vi "Write.vi"(8 "error in":errorcluster, 9 "Producer Ch":T2, 10 "Producer Control":T1, 11 "Cycler Cluster.lvclass":refnum<class "Power Supply Cluster.lvclass">) -> (0 "error out":errorcluster, 3 "output cluster":refnum<class "Power Supply Cluster.lvclass">)   [LabVIEW 2023, in "Power Supply Cluster.lvclass"]
uses:
  Power Supply Cluster.lvclass
  6bfc6677-cd67-4f2d-afef-839dec9218ce.vi
  74f11eb1-9425-41af-a169-6608e4aa6674.vi
  Producer Ch Array.ctl
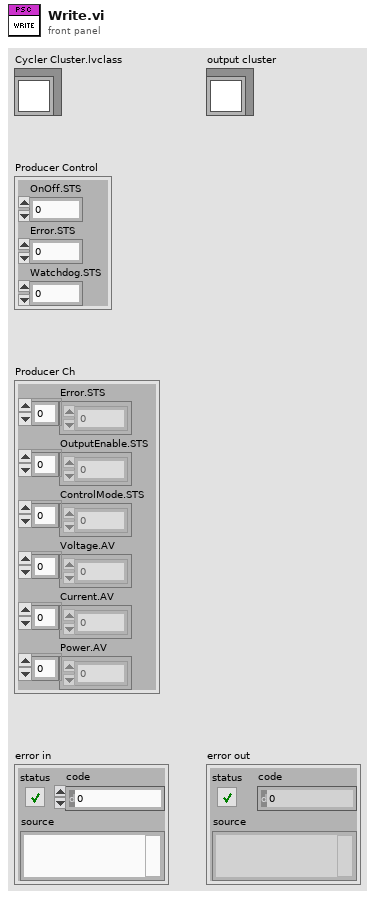
[diagram p1: front panel]
types:
  T1 = cluster{"OnOff.STS":i32, "Error.STS":i32, "Watchdog.STS":i32}
  T2 = typedef "Power Supply Cluster.lvclass/Producer Ch Array.ctl" = cluster{"Error.STS":i32[], "OutputEnable.STS":i32[], "ControlMode.STS":u16[], "Voltage.AV":dbl[], "Current.AV":dbl[], "Power.AV":dbl[]}
  T3 = cluster{"Error.STS":i32, "OutputEnable.STS":i32, "ControlMode.STS":u16, "Voltage.AV":dbl, "Current.AV":dbl, "Power.AV":dbl}
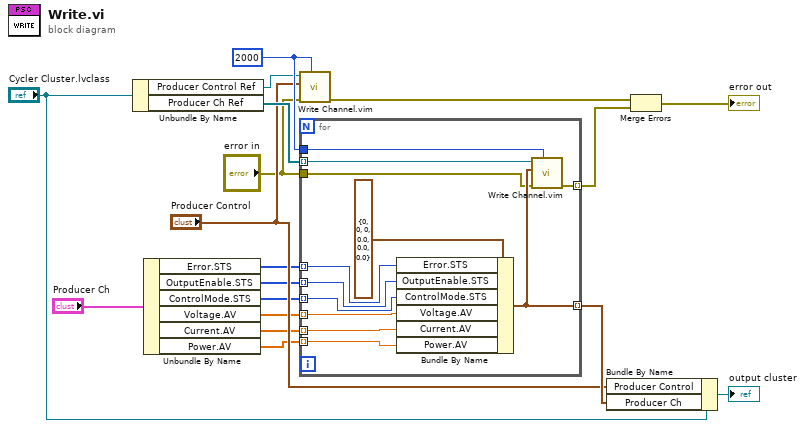
[diagram p0: block diagram]
diagram:
  w14 = 2000 ("Timeout (ms)")
  n1 = Unbundle By Name("Cycler Cluster.lvclass") -> ("Producer Control Ref"=w13:refnum<k21>, "Producer Ch Ref"=w15:refnum<k21>[])
  n2 = Unbundle By Name("Producer Ch") -> ("Error.STS"=w6:i32[], "OutputEnable.STS"=w5:i32[], "ControlMode.STS"=w4:u16[], "Voltage.AV"=w3:dbl[], "Current.AV"=w2:dbl[], "Power.AV"=w1:dbl[])
  n3 = call "Write Channel.vim"("Timeout (ms)"=w14, "error in"="error in", "Data in"="Producer Control", "ADAS HIL Channel in"=w13) -> ("error out"=w9:errorcluster)  [unwired: 5 in, 2 out]
  n4 = for {
    tunnel: [w29] -> w12 mode=indexing
    tunnel: "error in" -> [w28]
    tunnel: [w27] -> w8 mode=indexing
    tunnel: w15 -> [w26] mode=indexing
    tunnel: w14 -> [w25]
    tunnel: w6 -> [w24] mode=indexing
    tunnel: w5 -> [w23] mode=indexing
    tunnel: w4 -> [w22] mode=indexing
    tunnel: w3 -> [w21] mode=indexing
    tunnel: w2 -> [w20] mode=indexing
    tunnel: w1 -> [w19] mode=indexing
    n5 = Bundle By Name(cluster=T3 {"Error.STS"=0, "OutputEnable.STS"=0, "ControlMode.STS"=0, "Voltage.AV"=0.0, "Current.AV"=0.0, "Power.AV"=0.0} ("Producer Ch"), "Error.STS"=w24, "OutputEnable.STS"=w23, "ControlMode.STS"=w22, "Voltage.AV"=w21, "Current.AV"=w20, "Power.AV"=w19) -> (w29:T3)
    n6 = call "Write Channel.vim"("Timeout (ms)"=w25, "error in"=w28, "Data in"=w29, "ADAS HIL Channel in"=w26) -> ("error out"=w27:errorcluster)  [unwired: 5 in, 2 out]
  }
  n7 = Bundle By Name(cluster="Cycler Cluster.lvclass", "Producer Control"="Producer Control", "Producer Ch"=w12) -> (→"output cluster":refnum<class "Power Supply Cluster.lvclass">)
  n8 = Merge Errors(w9, w8) -> (→"error out":errorcluster)
